vi "height_sensor_equation_check.vi"() -> (8 "drone_lifting?":bool, 15 "Sensor_inserted?":bool)   [LabVIEW 2019]
uses:
  <vilib>/myRIO/Instrument Drivers/Onboard Devices/Accelerometer/typedefs/Accelerometer Reference.ctl
  <vilib>/myRIO/Common/Instrument Driver Framework/Utilities/typedefs/myRIO Generic Hardware Reference.ctl
  <vilib>/myRIO/Common/Instrument Driver Framework/Utilities/typedefs/Hardware Version Enum.ctl
  <vilib>/myRIO/Common/Instrument Driver Framework/Utilities/typedefs/myRIO v1.0 Reference.ctl
  <vilib>/myRIO/Common/Instrument Driver Framework/Utilities/typedefs/Generic FPGA Reference.ctl
  <vilib>/myRIO/Common/Instrument Driver Framework/myRIO v1.0/Accelerometer/typedefs/Accelerometer Channels List.ctl
  <vilib>/myRIO/Common/Instrument Driver Framework/myRIO v1.0/Accelerometer/typedefs/Accelerometer Channels Enum.ctl
  <vilib>/userdefined/High Color/nirio_resource_hc.ctl
  <vilib>/myRIO/Instrument Drivers/Onboard IO/AI/typedefs/AI Reference.ctl
  <vilib>/myRIO/Common/Instrument Driver Framework/myRIO v1.0/AI/typedefs/AI Channels List.ctl
  <vilib>/myRIO/Common/Instrument Driver Framework/myRIO v1.0/AI/typedefs/AI Channels Enum.ctl
  <vilib>/myRIO/Common/Instrument Driver Framework/Utilities/typedefs/Analog Scaling Constants List.ctl
  <vilib>/myRIO/Common/Instrument Driver Framework/Utilities/typedefs/Analog Scaling Constants.ctl
  <vilib>/myRIO/Instrument Drivers/Onboard IO/DIO/typedefs/DIO Reference.ctl
  <vilib>/myRIO/Common/Instrument Driver Framework/myRIO v1.0/DIO/typedefs/DIO Channels List.ctl
  <vilib>/myRIO/Common/Instrument Driver Framework/myRIO v1.0/DIO/typedefs/DIO Channels Enum.ctl
  <vilib>/myRIO/Common/Instrument Driver Framework/Utilities/vis/Is FPGA Ref Available.vi
  <vilib>/myRIO/Common/Instrument Driver Framework/myRIO v1.0/AI/vis/myRIO v1.1 Open AI.vi
  <vilib>/myRIO/Instrument Drivers/Onboard IO/AI/vis/Read.vi
  <vilib>/myRIO/Common/Instrument Driver Framework/myRIO v1.0/DIO/vis/myRIO v1.1 Open DIO.vi
  <vilib>/myRIO/Instrument Drivers/Onboard IO/DIO/vis/Read.vi
  <vilib>/myRIO/Common/Instrument Driver Framework/myRIO v1.0/Accelerometer/vis/myRIO v1.1 Open Accelerometer.vi
  <vilib>/myRIO/Instrument Drivers/Onboard Devices/Accelerometer/vis/Read.vi
  <vilib>/myRIO/Common/Instrument Driver Framework/Utilities/vis/Validate Channels.vi
  <vilib>/myRIO/Common/Instrument Driver Framework/myRIO v1.0/AI/vis/myRIO v1.0 Reserve AI.vi
  <vilib>/myRIO/Common/Instrument Driver Framework/myRIO v1.0/DIO/vis/myRIO v1.0 Reserve DIO.vi
  <vilib>/myRIO/Common/Instrument Driver Framework/myRIO v1.0/Accelerometer/vis/myRIO v1.0 Reserve Accelerometer.vi
  <vilib>/myRIO/Common/Instrument Driver Framework/myRIO v1.0/AI/vis/myRIO v1.0 Build MUX Configuration AI.vi
  <vilib>/myRIO/Common/Instrument Driver Framework/myRIO v1.0/Resource Manager/vis/myRIO v1.0 Reserve Channel List.vi
  <vilib>/myRIO/Common/Instrument Driver Framework/myRIO v1.0/DIO/vis/myRIO v1.0 Build MUX Configuration DIO.vi
  <vilib>/myRIO/Common/Instrument Driver Framework/myRIO v1.0/Accelerometer/vis/myRIO v1.0 Build MUX Configuration Accelerometer.vi
  <vilib>/myRIO/Common/Instrument Driver Framework/myRIO v1.0/Resource Manager/vis/myRIO v1.0 Reserve Channel.vi
  <vilib>/myRIO/Common/Instrument Driver Framework/myRIO v1.0/Resource Manager/vis/myRIO v1.0 Unreserve Channel.vi
  <vilib>/myRIO/Common/Instrument Driver Framework/myRIO v1.0/Resource Manager/vis/myRIO v1.0 Create Configuration List.vi
  <vilib>/myRIO/Common/Instrument Driver Framework/myRIO v1.0/Resource Manager/vis/myRIO v1.0 Build Mutex Name.vi
  <vilib>/Utility/VariantDataType/GetNumericInfo.vi
  <vilib>/Utility/error.llb/Error Cluster From Error Code.vi
  <vilib>/myRIO/Common/Instrument Driver Framework/myRIO v1.0/myRIO v1.1 Open.vi
  <vilib>/myRIO/Common/Instrument Driver Framework/myRIO v1.0/Accelerometer/vis/myRIO v1.0 Get Scaling Constant Accelerometer.vi
  <vilib>/myRIO/Common/Instrument Driver Framework/Utilities/vis/IO Manager.vi
  <vilib>/myRIO/Common/Instrument Driver Framework/Utilities/vis/Configuration Manager.vi
  <vilib>/myRIO/Common/Instrument Driver Framework/myRIO v1.0/myRIO v1.0 Close.vi
  <vilib>/myRIO/Common/Instrument Driver Framework/myRIO v1.0/Accelerometer/vis/myRIO v1.0 Read Accelerometer.vi
  <vilib>/myRIO/Common/Instrument Driver Framework/myRIO v1.0/AI/vis/myRIO v1.0 Get Scaling Constants AI.vi
  <vilib>/myRIO/Common/Instrument Driver Framework/myRIO v1.0/AI/vis/myRIO v1.0 Read AI.vi
  <vilib>/myRIO/Common/Instrument Driver Framework/myRIO v1.0/Resource Manager/vis/myRIO v1.0 Configure IO.vi
  <vilib>/myRIO/Common/Instrument Driver Framework/myRIO v1.0/DIO/vis/myRIO v1.0 Read DIO.vi
  <vilib>/Utility/file.llb/Write Delimited Spreadsheet (DBL).vi
  <vilib>/myRIO/Express VI/Onboard Devices/Accelerometer/Accelerometer Express VI.xnode
  <vilib>/myRIO/Instrument Drivers/Onboard Devices/Accelerometer/vis/myRIO Accelerometer Open.xnode
  <vilib>/myRIO/Express VI/Onboard IO/AI/AI Express VI.xnode
  <vilib>/myRIO/Instrument Drivers/Onboard IO/AI/vis/myRIO AI Open.xnode
  <vilib>/myRIO/Express VI/Onboard IO/DI/DI Express VI.xnode
  <vilib>/myRIO/Instrument Drivers/Onboard IO/DIO/vis/myRIO DIO Open.xnode
  <vilib>/myRIO/Instrument Drivers/Onboard Devices/Accelerometer/Accelerometer.lvlib
  <vilib>/myRIO/Instrument Drivers/Onboard IO/AI/AI.lvlib
  <vilib>/myRIO/Instrument Drivers/Onboard IO/DIO/DIO.lvlib
panel:
  out "LP_avg":dbl
  out "LP_threshold":dbl
  out "Time in seconds":i32
  out "sensor_ideal_count":i32
  out "height_difference":dbl
  out "height":dbl
  out "Potentiometer":dbl
  out "change_in_x_axis":dbl
  out "change_in_z_axis":dbl
  out "z-axis_acc_data":dbl
  out "x-axis_acc_Data":dbl
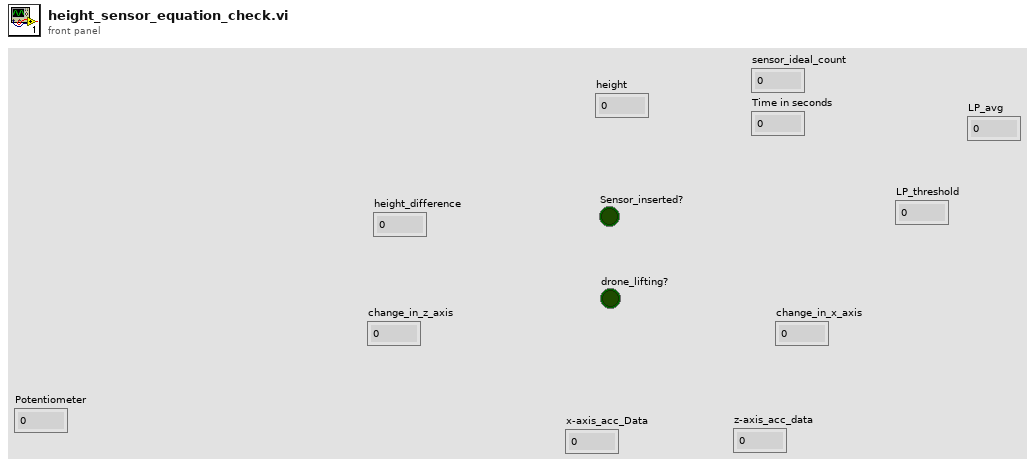
[diagram p1: front panel]
types:
  T1 = typedef "AI.lvlib/AI Reference.ctl" = cluster{"myRIO Reference":T2, "AI Channels List":T6, "AI Scaling Constants List":T8}
  T2 = typedef "myRIO Generic Hardware Reference.ctl" = cluster{"myRIO Model":T3, "myRIO Hardware Reference":T4}
  T3 = typedef "Hardware Version Enum.ctl" = enum16{"Unknown", "myRIO-1900", "myRIO-1950", "roboRIO", "NI ELVIS RIO CM", "ELVIS III"}
  T4 = typedef "myRIO v1.0 Reference.ctl" = cluster{"Generic FPGA Reference":T5, "Allow multiple opens":bool}
  T5 = typedef "Generic FPGA Reference.ctl" = refnum<k20>
  T6 = typedef "AI Channels List.ctl" = T7[]
  T7 = typedef "AI Channels Enum.ctl" = enum16{"Not Connected", "AudioIn/Left", "AudioIn/Right", "C/AI0", "C/AI1", "A/AI0", "A/AI1", "A/AI2", "A/AI3", "A/AI4", "A/AI5", "A/AI6", "A/AI7", "B/AI0", "B/AI1", "B/AI2", "B/AI3", "B/AI4", "B/AI5", "B/AI6", "B/AI7", "AI/AI0", "AI/AI1", "AI/AI2", "AI/AI3", "A/AI0 (DIFF)", "A/AI1 (DIFF)", "A/AI2 (DIFF)", "A/AI3 (DIFF)", "B/AI0 (DIFF)", "B/AI1 (DIFF)", "B/AI2 (DIFF)", "B/AI3 (DIFF)"}
  T8 = typedef "Analog Scaling Constants List.ctl" = T9[]
  T9 = typedef "Analog Scaling Constants.ctl" = cluster{"LSB Weight (Volts)":dbl, "Offset (Volts)":dbl, "Signed?":bool}
  T10 = typedef "nirio_resource_hc.ctl" = tag
  T11 = typedef "DIO.lvlib/DIO Reference.ctl" = cluster{"myRIO Reference":T2, "DIO Channels List":T12}
  T12 = typedef "DIO Channels List.ctl" = T13[]
  T13 = typedef "DIO Channels Enum.ctl" = enum16{"Not Connected", "C/DIO0", "C/DIO1", "C/DIO2", "C/DIO3", "C/DIO4", "C/DIO5", "C/DIO6", "C/DIO7", "A/DIO0", "A/DIO1", "A/DIO2", "A/DIO3", "A/DIO4", "A/DIO5", "A/DIO6", "A/DIO7", "A/DIO8", "A/DIO9", "A/DIO10", "A/DIO11", "A/DIO12", "A/DIO13", "A/DIO14", "A/DIO15", "A/DIO16", "A/DIO17", "A/DIO18", "A/DIO19", "B/DIO0", "B/DIO1", "B/DIO2", "B/DIO3", "B/DIO4", "B/DIO5", "B/DIO6", "B/DIO7", "B/DIO8", "B/DIO9", "B/DIO10", "B/DIO11", "B/DIO12", "B/DIO13", "B/DIO14", "B/DIO15", "B/DIO16", "B/DIO17", "B/DIO18", "B/DIO19", "LED0", "LED1", "LED2", "LED3", "Button0", "DIO/DIO0", "DIO/DIO1", "DIO/DIO2", "DIO/DIO3", "DIO/DIO4", "DIO/DIO5", "DIO/DIO6", "DIO/DIO7", "DIO/DIO8", "DIO/DIO9", "SPI/CS0", "SPI/CS1", "SPI/CS2", "SPI/CS3", "LED RADIO (Green)", "LED RADIO (Red)", "LED COMM (Green)", "LED COMM (Red)", "LED MODE (Green)", "LED MODE (Red)"}
  T14 = typedef "Accelerometer.lvlib/Accelerometer Reference.ctl" = cluster{"myRIO Reference":T2, "Accelerometer Channels List":T15, "LSB Weight":dbl}
  T15 = typedef "Accelerometer Channels List.ctl" = T16[]
  T16 = typedef "Accelerometer Channels Enum.ctl" = enum16{"Not Connected", "X-Axis", "Y-Axis", "Z-Axis"}
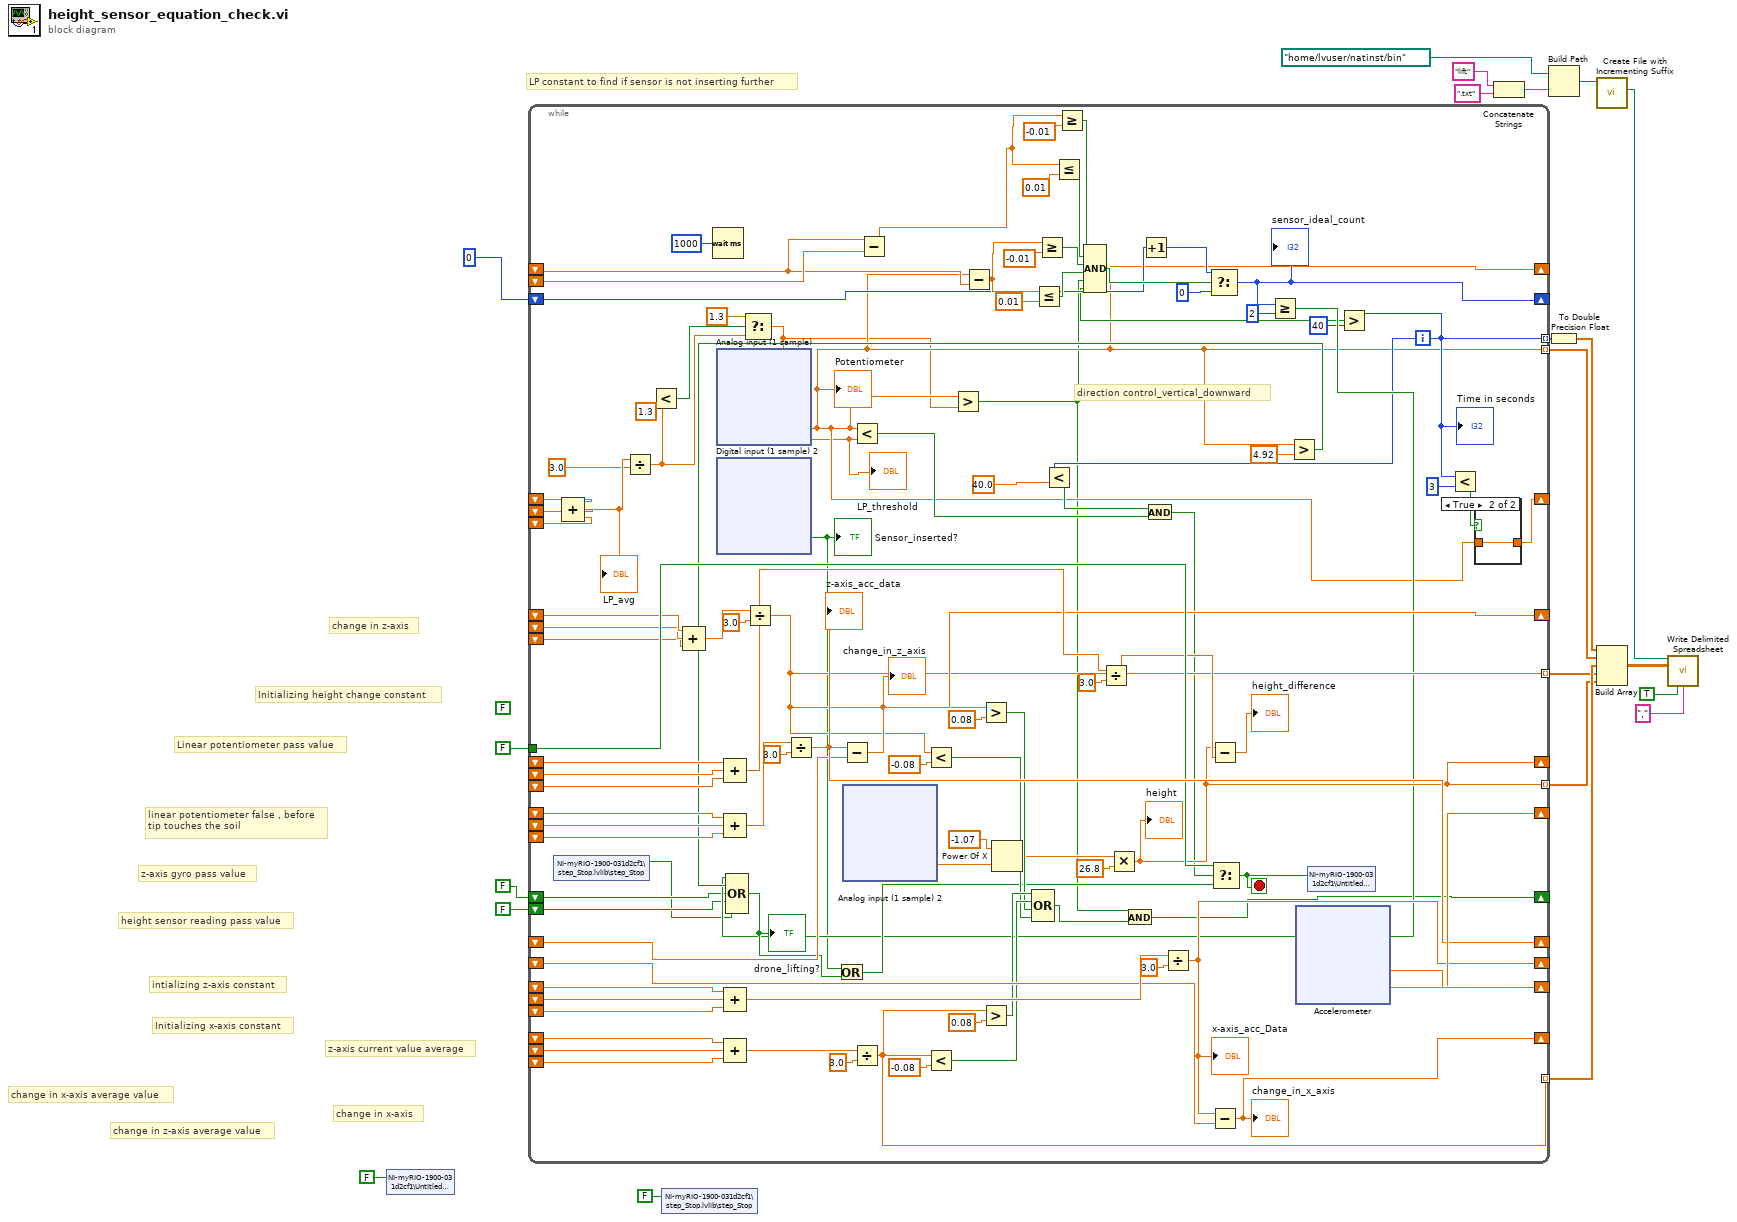
[diagram p0: block diagram]
diagram:
  (unwired) FALSE
  # "LP constant to find if sensor is not inserting further"
  # "change in z-axis average value"
  # "change in x-axis average value"
  # "change in x-axis"
  # "z-axis current value average"
  # "Initializing x-axis constant"
  # "intializing z-axis constant"
  # "height sensor reading pass value"
  # "z-axis gyro pass value"
  # "Linear potentiometer pass value"
  # "Initializing height change constant"
  # "linear potentiometer false , before\ntip touches the soil"
  # "change in z-axis"
  n1 = shared-variable "NI-myRIO-1900-031d2cf1\\Untitled Library 1.lvlib\\stop"(FALSE ("stop")) -> ()  [unwired: 1 in, 1 out]
  n2 = while {
    shift-right: [w125] -> _
    shift-left: _ -> [w122]
    shift-left: _ -> [w123]
    shift-left: _ -> [w124]
    shift-right: [w115] -> _
    shift-left: _ -> [w116]
    shift-left: _ -> [w117]
    shift-left: _ -> [w118]
    shift-right: [w113] -> _
    shift-left: _ -> [w112]
    shift-right: [w107] -> _
    shift-left: _ -> [w106]
    tunnel: [w30] -> w14 mode=indexing
    tunnel: [w78] -> w13 mode=indexing
    tunnel: [w71] -> w12 mode=indexing
    shift-right: [w23] -> _
    shift-left: FALSE -> [w50]
    shift-left: FALSE -> [w49]
    tunnel: FALSE -> [w100]
    shift-right: [w86] -> _
    shift-left: _ -> [w89]
    shift-left: _ -> [w88]
    shift-left: _ -> [w87]
    tunnel: [w86] -> w8 mode=indexing
    shift-right: [w79] -> _
    shift-left: _ -> [w82]
    shift-left: _ -> [w83]
    shift-left: _ -> [w84]
    tunnel: [w34] -> w6 mode=indexing
    shift-right: [w77] -> _
    shift-left: _ -> [w74]
    shift-left: _ -> [w73]
    shift-left: _ -> [w72]
    shift-right: [w30] -> _
    shift-left: _ -> [w56]
    shift-right: [w60] -> _
    shift-left: 0 -> [w61]
    shift-left: _ -> [w57]
    shift-right: [w31] -> _
    shift-left: _ -> [w39]
    shift-left: _ -> [w38]
    shift-left: _ -> [w37]
    i -> [w34]
    stop <- w98 stop-if-true
    # "direction control_vertical_downward"
    n3 = shared-variable "NI-myRIO-1900-031d2cf1\\step_Stop.lvlib\\step_Stop"() -> (w44:bool)  [unwired: 1 in, 1 out]
    n4 = Compound Arithmetic op=ADD(w39, w38, w37) -> (w36:dbl)
    "LP_avg" <- w36
    n5 = Divide(x=w36, y=3.0) -> (x/y=w26:dbl)
    n6 = Less?(x=w26, y=1.3) -> (x < y?=w28:bool)
    n7 = Compound Arithmetic op=ADD(w74, w73, w72) -> (w75:dbl)
    n8 = Wait (ms)(milliseconds to wait=u32 1000) -> ()  [unwired: 1 out]
    n9 = xnode "Analog input (1 sample)"() -> ("A/AI0 (Pin 3)"=w30:dbl)  [unwired: 1 in, 1 out]
    "Potentiometer" <- w30
    n10 = xnode "Digital input (1 sample) 2"() -> ("C/DIO5 (DIO5)"=w48:bool)  [unwired: 1 in, 1 out]
    "Sensor_inserted?" <- w48
    n11 = Compound Arithmetic op=ADD(w89, w88, w87) -> (w92:dbl)
    n12 = Compound Arithmetic op=ADD(w116, w117, w118) -> (w119:dbl)
    n13 = Compound Arithmetic op=ADD(w122, w123, w124) -> (w121:dbl)
    n14 = Compound Arithmetic op=ADD(w84, w83, w82) -> (w80:dbl)
    n15 = Select(t=1.3, s=w28, f=w26) -> (s? t:f=w25:dbl)
    "LP_threshold" <- w25
    n16 = Divide(x=w75, y=3.0) -> (x/y=w71:dbl)
    n17 = Divide(x=w119, y=3.0) -> (x/y=w113:dbl)
    "z-axis_acc_data" <- w113
    n18 = Subtract(x=w113, y=w112) -> (x-y=w77:dbl)
    "change_in_z_axis" <- w77
    n19 = xnode "Analog input (1 sample) 2"() -> ("B/AI1 (Pin 5)"=w94:dbl)  [unwired: 1 in, 1 out]
    n20 = Less?(x=w30, y=w25) -> (x < y?=w41:bool)
    n21 = Divide(x=w80, y=3.0) -> (x/y=w78:dbl)
    n22 = Subtract(x=w56, y=w57) -> (x-y=w53:dbl)
    n23 = Less?(x=w71, y=-0.08) -> (x < y?=w102:bool)
    n24 = Less?(x=w78, y=-0.08) -> (x < y?=w104:bool)
    n25 = Greater?(x=w30, y=w25) -> (0:w22:bool)
    n26 = Subtract(x=w30, y=w56) -> (x-y=w67:dbl)
    n27 = Greater?(x=w71, y=0.08) -> (0:w103:bool)
    n28 = Greater?(x=w78, y=0.08) -> (0:w105:bool)
    n29 = Power Of X(1:w94, 2:-1.07 ("y")) -> (0:w96:dbl)
    n30 = Compound Arithmetic op=OR(w105, w104, w103, w102) -> (w24:bool)
    n31 = Less Or Equal?(x=w67, y=0.01) -> (x <= y?=w64:bool)
    n32 = Greater Or Equal?(x=w67, y=-0.01) -> (x >= y?=w65:bool)
    n33 = Less?(x=w34, y=40.0) -> (x < y?=w42:bool)
    n34 = Less Or Equal?(x=w53, y=0.01) -> (x <= y?=w52:bool)
    n35 = Greater Or Equal?(x=w53, y=-0.01) -> (x >= y?=w51:bool)
    n36 = Divide(x=w92, y=3.0) -> (x/y=w90:dbl)
    n37 = Multiply(x=w96, y=26.8) -> (x*y=w86:dbl)
    "height" <- w86
    n38 = And(x=w22, y=w24) -> (x .and. y?=w23:bool)
    n39 = Increment(x=w61) -> (x+1=w62:i32)
    n40 = And(x=w42, y=w41) -> (x .and. y?=w40:bool)
    n41 = Divide(x=w121, y=3.0) -> (x/y=w107:dbl)
    "x-axis_acc_Data" <- w107
    n42 = Subtract(x=w86, y=w90) -> (x-y=→"height_difference":dbl)
    n43 = Subtract(x=w107, y=w106) -> (x-y=w79:dbl)
    "change_in_x_axis" <- w79
    n44 = Greater?(x=w30, y=4.92) -> (0:w69:bool)
    n45 = xnode "Accelerometer"() -> ("X-Axis"=w125:dbl, "Z-Axis"=w115:dbl)  [unwired: 1 in, 1 out]
    n46 = Greater?(x=w34, y=40) -> (0:w45:bool)
    n47 = Compound Arithmetic op=AND(w51, w52, w65, w64, w22, w45) -> (w63:bool)
    n48 = Select(t=w62, s=w63, f=0) -> (s? t:f=w60:i32)
    "sensor_ideal_count" <- w60
    n49 = Greater Or Equal?(x=w60, y=2) -> (x >= y?=w58:bool)
    n50 = Compound Arithmetic op=OR(w58, w69, w50, w49, w44) -> (w101:bool)
    "drone_lifting?" <- w101
    n51 = Or(x=w48, y=w101) -> (x .or. y?=w99:bool)
    n52 = Select(t=w100, s=w40, f=w99) -> (s? t:f=w98:bool)
    n53 = shared-variable "NI-myRIO-1900-031d2cf1\\Untitled Library 1.lvlib\\stop"(w98) -> ()  [unwired: 1 in, 1 out]
    n54 = Less?(x=w34, y=3) -> (x < y?=w32:bool)
    n55 = case shown="True" w32 {
      tunnel: w30 -> [_ w126]
      tunnel: [_ w126] -> w31
      frame False {
      }
      frame True {
      }
    }
    "Time in seconds" <- w34
  }
  n56 = shared-variable "NI-myRIO-1900-031d2cf1\\step_Stop.lvlib\\step_Stop"(FALSE ("step_Stop")) -> ()  [unwired: 1 in, 1 out]
  n57 = Concatenate Strings("lift" ("string"), ".txt" ("string")) -> (w19:string)
  n58 = Build Path(base path=path "/home/lvuser/natinst/bin", name or relative path=w19) -> (appended path=w15:path)
  n59 = To Double Precision Float(number=w6) -> (double precision float=w5:dbl[])
  n60 = call <vilib>:"Create File with Incrementing Suffix.vi"("file path"=w15) -> ("actual path"=w3:path)  [unwired: 8 in, 2 out]
  n61 = Build Array(w5, w14, w13, w12, w8) -> (w2:dbl[][])
  n62 = call-poly <vilib>:"Write Delimited Spreadsheet.vi"("file path (dialog if empty)"=w3, "2D data"=w2, "transpose? (no:F)"=TRUE, "delimiter (\\t)"="," ("delimiter (\\t)")) -> ()  [unwired: 10 in, 2 out]
